vi "Select User Info.vi"(8 "error in (no error)":errorcluster, 10 "Current Account":string, 11 "DBlink":string="Driver={ODBC Driver 17 for SQL Server};Server=localhost\\SQLEXPRESS;Database=ZDX201;UID=labview;PWD=Dsa@54137926") -> (0 "error out":errorcluster, 2 "user info":T1)   [LabVIEW 2019]
uses:
  <vilib>/addons/database/Connection.llb/DB Tools Open Connec (String).vi
  <vilib>/addons/database/_DB Variant To Data/Database Variant To Data.xnode
  <vilib>/addons/database/NI_Database_API.lvlib
panel:
  in  "columns":string[](array[string])=["account", "password", "authority"]
  in  "user info":T2(array[cluster])
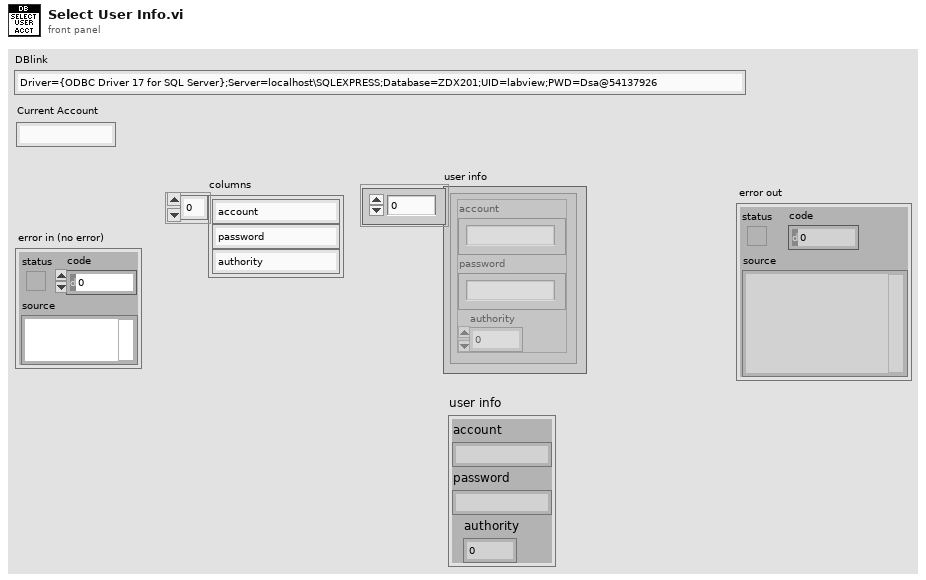
[diagram p1: front panel]
types:
  T1 = cluster{"account":string, "password":string, "authority":i32}
  T2 = cluster{"account":string, "password":string, "authority":i32}[]
  T3 = typedef "NI_Database_API.lvlib/Conn ObjectReference.ctl" = refnum<k1>
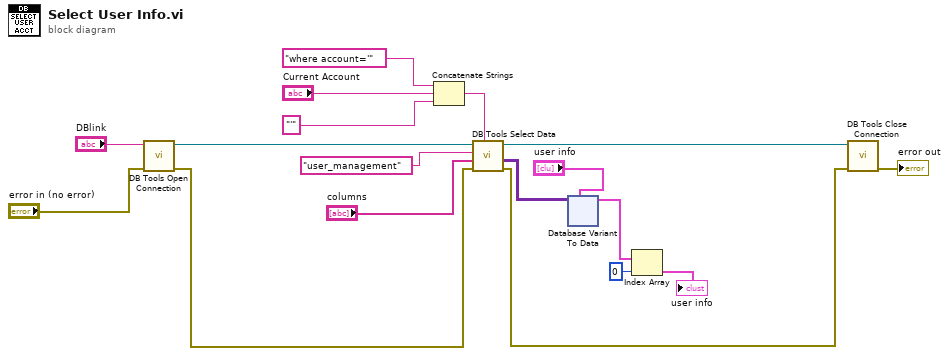
[diagram p0: block diagram]
diagram:
  n1 = call-poly <vilib>:"DB Tools Open Connection.vi"("error in (no error)"="error in (no error)", "connection information"="DBlink") -> ("error out"=w13:errorcluster, "connection reference"=w14:T3)  [unwired: 6 in]
  n2 = Concatenate Strings("where account='" ("format string"), "Current Account", "'" ("format string")) -> (w5:string)
  n3 = call <vilib>:"DB Tools Select Data.vi"("condition"=w5, "error in (no error)"=w13, "columns"="columns", "table"="user_management", "connection reference"=w14) -> ("error out"=w10:errorcluster, "data"=w18:variant[][], "connection reference out"=w11:T3)  [unwired: 1 in]
  n4 = xnode "Database Variant To Data"("database variant"=w18, "type"="user info") -> ("data"=w4:T2)  [unwired: 1 in, 1 out]
  n5 = Index Array(array=w4, index=0) -> (element=→"user info":T1)
  n6 = call <vilib>:"DB Tools Close Connection.vi"("error in (no error)"=w10, "connection reference"=w11) -> ("error out"=→"error out":errorcluster)  [unwired: 5 in]
